vi "日期键盘.vi"(11 "原值":string) -> (3 "x+y":string)   [LabVIEW 2016, in "数据查询.lvlib"]
uses:
  <vilib>/Utility/miscctls.llb/LVPointTypeDef.ctl
panel:
  in  "日":string(combo)="01"
  in  "月":string(combo)="01"
  in  "年":string(combo)="2000"
  in  "取消按钮":bool
  in  "停止":bool
  # "年"
  # "月"
  # "日"
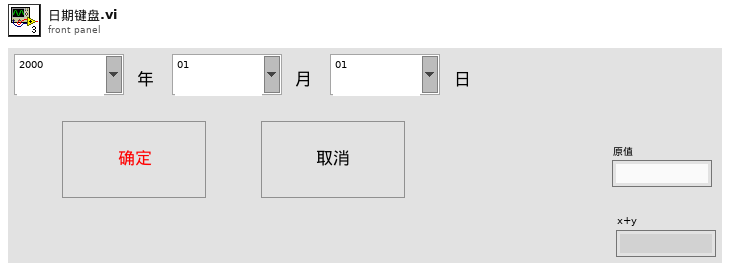
[diagram p1: front panel]
types:
  T1 = typedef "LVPointTypeDef.ctl" = cluster{"Horizontal":i16, "Vertical":i16}
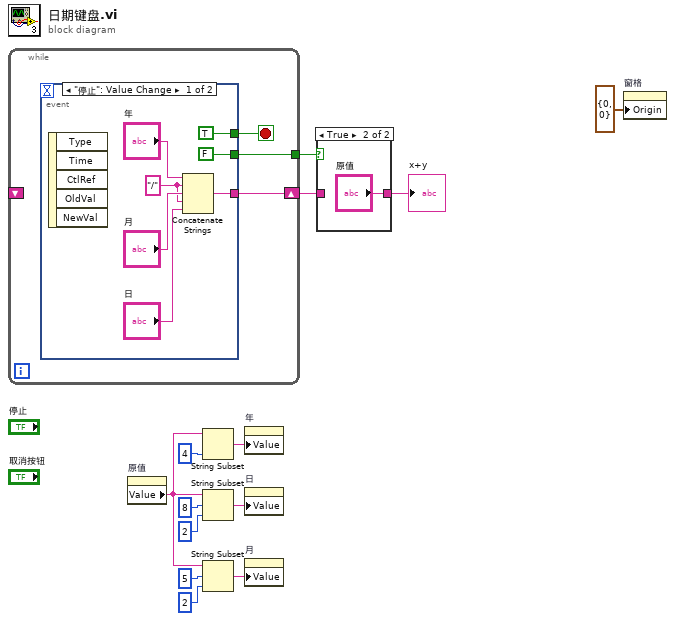
[diagram p0: block diagram]
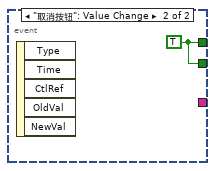
[diagram p3: hidden frame]
diagram:
  n1 = while {
    shift-right: [w14] -> w13
    shift-left: _ -> [_]
    tunnel: [w15] -> w11
    stop <- w16 stop-if-true
    n2 = event shown="[0] \"停止\": Value Change" {
      selector: _ -> [_ _]
      dyn-events: _ -> [_ _]
      timeout: _ -> [_ _]
      tunnel: [TRUE w24] -> w16
      tunnel: [w17 _] -> w14
      tunnel: [FALSE w24] -> w15
      event "停止": Value Change {
        w18 = "/" ("字符串")
        n3 = event-data() -> ()  [unwired: 1 in, 5 out]
        n4 = Concatenate Strings("年", w18, "月", w18, "日") -> (w17:string)
      }
      event "取消按钮": Value Change {
        w24 = TRUE
        n5 = event-data() -> ()  [unwired: 1 in, 5 out]
      }
    }
  }
  n6 = property on="原值" class="Str"() -> ("Value"=w5:string)  [unwired: 2 in, 2 out]
  n7 = String Subset(string=w5, length (rest)=4 ("长度（剩余）")) -> (substring=w8:string)  [unwired: 1 in]
  n8 = String Subset(string=w5, offset (0)=8 ("偏移量(0)"), length (rest)=2 ("长度（剩余）")) -> (substring=w1:string)
  n9 = String Subset(string=w5, offset (0)=5 ("偏移量(0)"), length (rest)=2 ("长度（剩余）")) -> (substring=w2:string)
  n10 = property on="年" class="CmbBox"("Value"=w8) -> ()  [unwired: 2 in, 2 out]
  n11 = property on="日" class="CmbBox"("Value"=w1) -> ()  [unwired: 2 in, 2 out]
  n12 = property on="月" class="CmbBox"("Value"=w2) -> ()  [unwired: 2 in, 2 out]
  n13 = case shown="True" w11 {
    tunnel: w13 -> [w25 _]
    tunnel: [w25 "原值"] -> w12
    frame False {
    }
    frame True {
    }
  }
  "x+y" <- w12
  n14 = property on="窗格" class="Pane"("Origin"=T1 {"Horizontal"=0, "Vertical"=0} ("原点")) -> ()  [unwired: 2 in, 2 out]
